vi "eval.vi"(8 "Environment in":T1, 9 "Expression in":T2) -> (2 "Environment out":T1, 3 "Expression out":T2)   [LabVIEW 2021]
uses:
  Expression.ctl
  ExpressionType.ctl
  Environment.ctl
  ClosureData.ctl
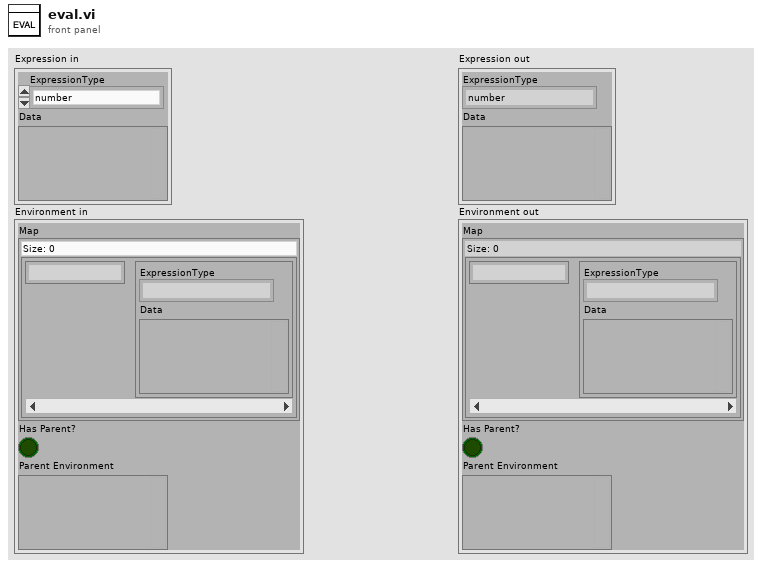
[diagram p1: front panel]
types:
  T1 = typedef "Environment.ctl" = cluster{"Map":map{string, T2}, "Has Parent?":bool, "Parent Environment":variant}
  T2 = typedef "Expression.ctl" = cluster{"ExpressionType":T3, "Data":variant}
  T3 = typedef "ExpressionType.ctl" = enum16{"number", "string", "symbol", "primitive", "list", "closure", "nil", "error"}
  T4 = typedef "ClosureData.ctl" = cluster{"arguments":string[], "code":T2}
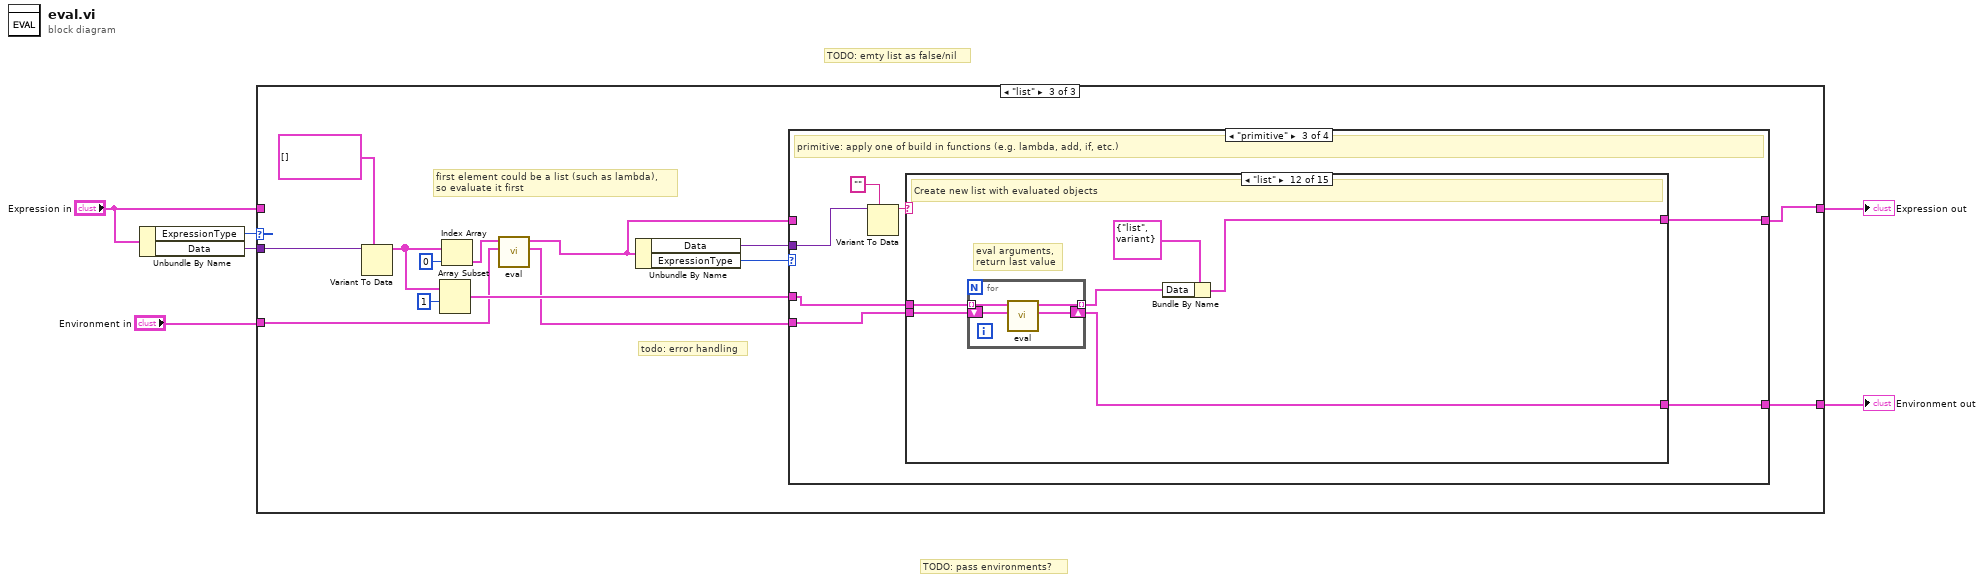
[diagram p0: block diagram]
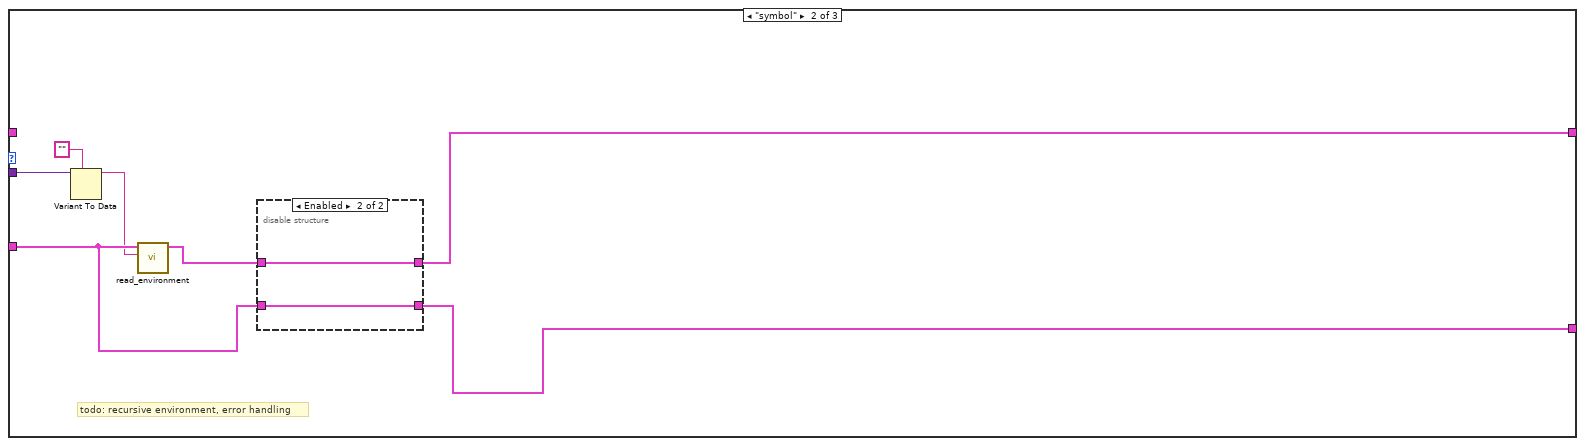
[diagram p3: hidden frame]
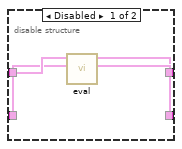
[diagram p4: hidden frame]
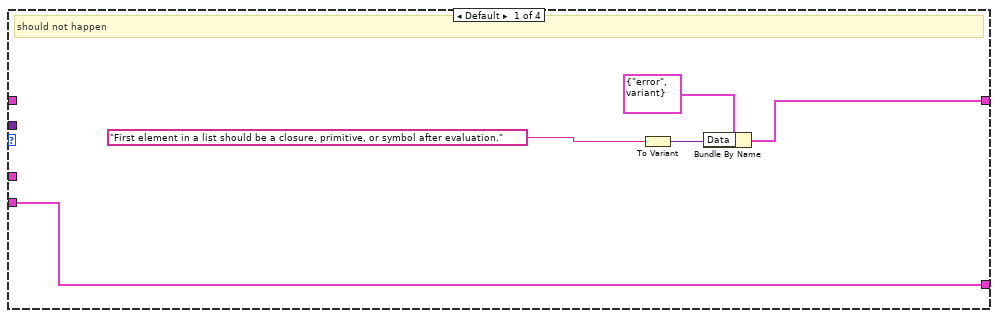
[diagram p5: hidden frame]
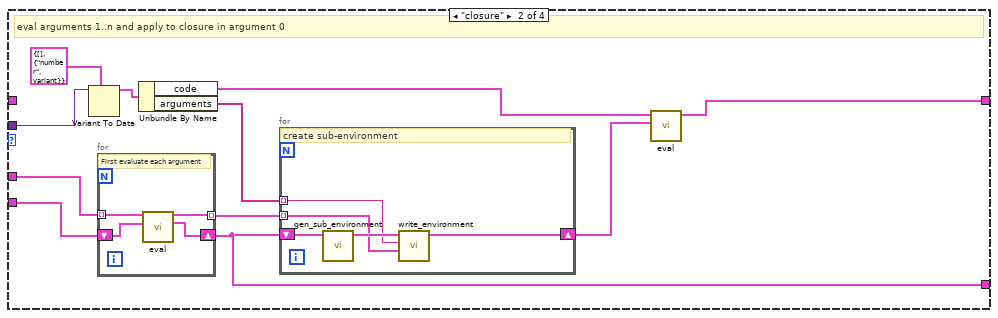
[diagram p6: hidden frame]
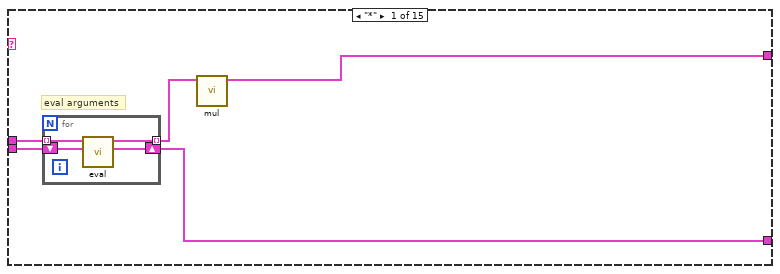
[diagram p7: hidden frame]
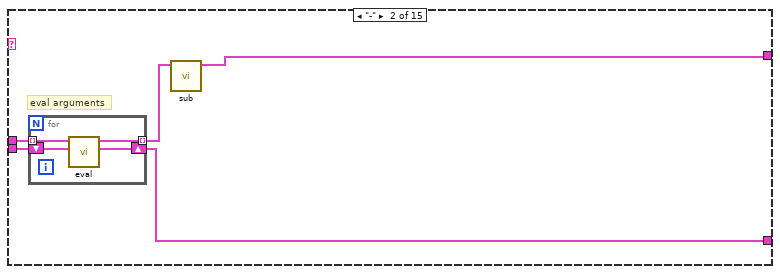
[diagram p8: hidden frame]
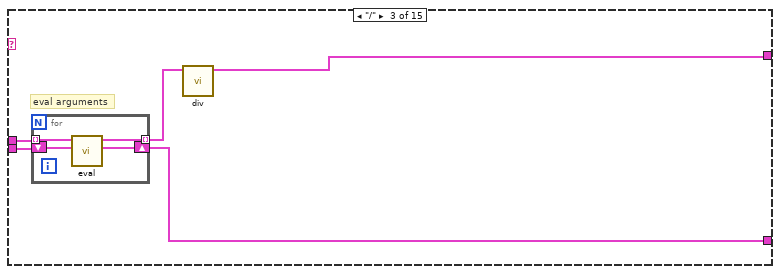
[diagram p9: hidden frame]
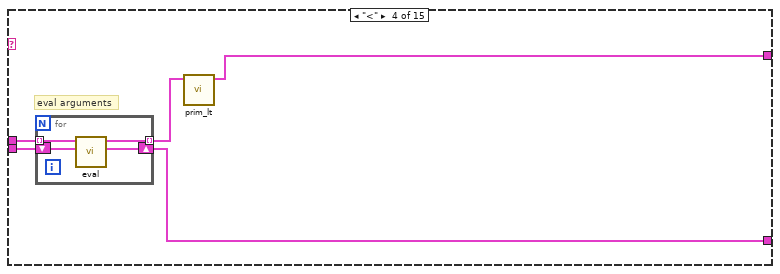
[diagram p10: hidden frame]
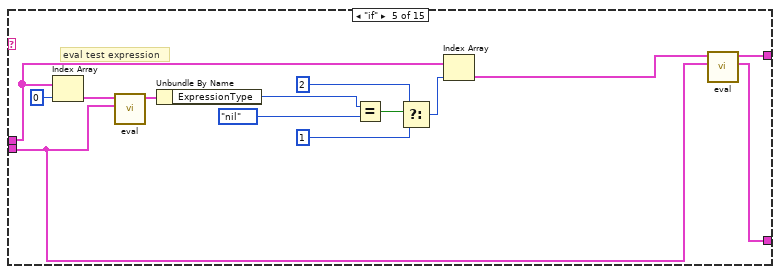
[diagram p11: hidden frame]
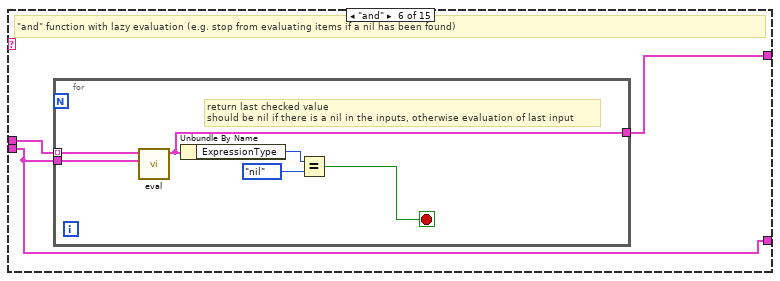
[diagram p12: hidden frame]
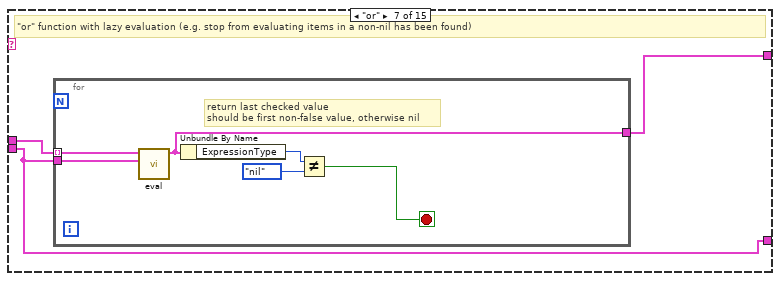
[diagram p13: hidden frame]
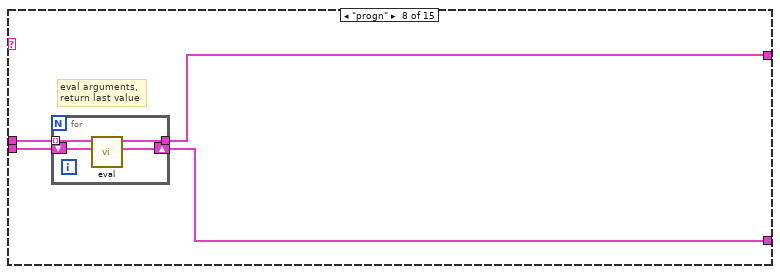
[diagram p14: hidden frame]
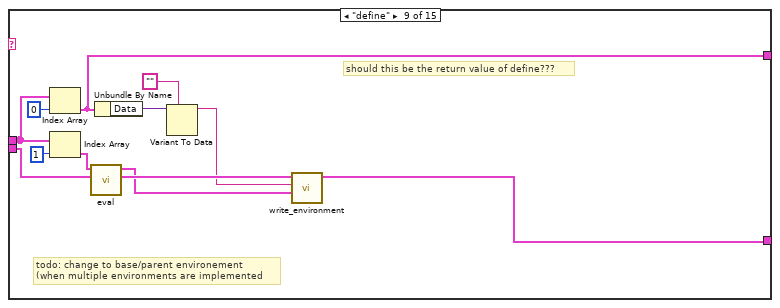
[diagram p15: hidden frame]
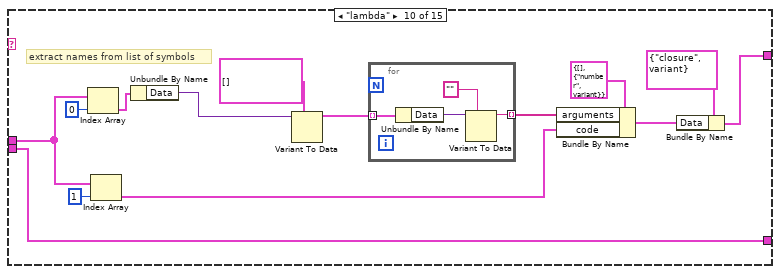
[diagram p16: hidden frame]
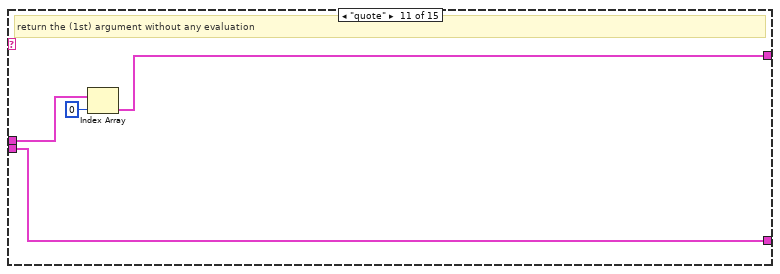
[diagram p17: hidden frame]
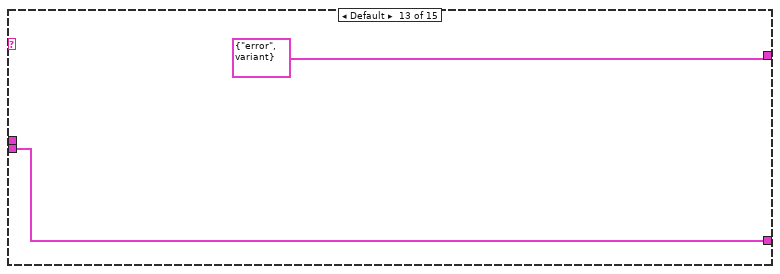
[diagram p18: hidden frame]
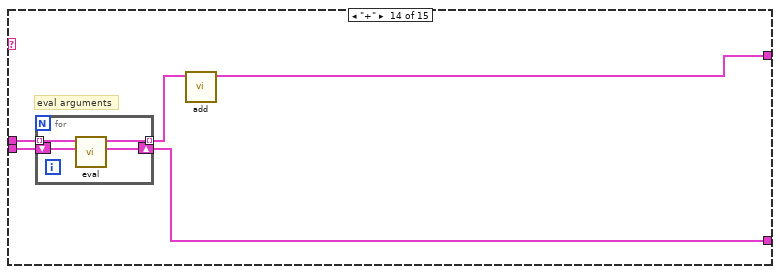
[diagram p19: hidden frame]
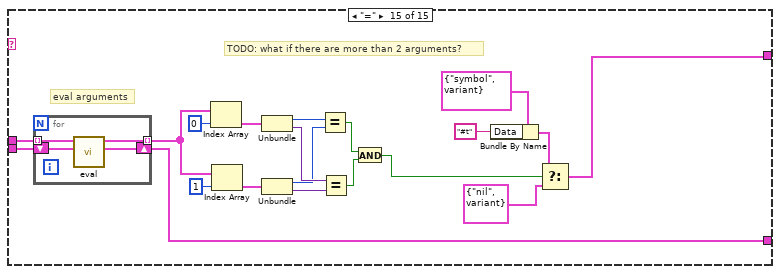
[diagram p20: hidden frame]
diagram:
  # "TODO: pass environments?"
  # "TODO: emty list as false/nil"
  n1 = Unbundle By Name("Expression in") -> ("ExpressionType"=w5:T3, "Data"=w3:variant)
  n2 = case shown="\"list\"" w5 {
    tunnel: "Expression in" -> [w8 _ _]
    tunnel: [w8 w12 w31] -> w4
    tunnel: "Environment in" -> [w7 w11 w23]
    tunnel: w3 -> [_ w15 w34]
    tunnel: [w7 w13 w22] -> w1
    frame "number", "string", "primitive", "closure".."error" {
    }
    frame "symbol" {
      # "todo: recursive environment, error handling"
      n3 = Variant To Data(type="", Variant=w15) -> (data=w9:string)  [unwired: 1 in, 1 out]
      n4 = call "read_environment.vi"("symbol"=w9, "Environment in"=w11) -> ("Expression"=w10:T2)  [unwired: 9 in]
      n5 = disable-structure shown="Enabled" {
        disable-tunnel: w10 -> [w19 w21]
        disable-tunnel: w11 -> [w18 w20]
        disable-tunnel: [w17 w20] -> w13
        disable-tunnel: [w16 w21] -> w12
        frame Disabled {
          n6 = call "eval.vi"("Environment in"=w18, "Expression in"=w19) -> ("Environment out"=w17:T1, "Expression out"=w16:T2)  [unwired: 6 in]
        }
        frame Enabled {
        }
      }
    }
    frame "list" {
      # "first element could be a list (such as lambda),\nso evaluate it first"
      # "todo: error handling"
      n7 = Variant To Data(type=T2[] [], Variant=w34) -> (data=w29:T2[])  [unwired: 1 in, 1 out]
      n8 = Array Subset(array=w29, index=1) -> (w28:T2[])  [unwired: 1 in]
      n9 = Index Array(array=w29, index=0) -> (element=w25:T2)
      n10 = call "eval.vi"("Environment in"=w23, "Expression in"=w25) -> ("Environment out"=w26:T1, "Expression out"=w24:T2)  [unwired: 6 in]
      n11 = Unbundle By Name(w24) -> ("Data"=w32:variant, "ExpressionType"=w27:T3)
      n12 = case shown="\"primitive\"" w27 {
        tunnel: w32 -> [_ w48 w66 w227]
        tunnel: w24 -> [_ _ _ _]
        tunnel: w26 -> [w40 w51 w62 w225]
        tunnel: [w36 w41 w64 w223] -> w31
        tunnel: w28 -> [_ w50 w63 _]
        tunnel: [w40 w44 w61 w225] -> w22
        frame Default {
          # "should not happen"
          n13 = To Variant(anything="First element in a list should be a closure, primitive, or symbol after evaluation.") -> (Variant=w38:variant)
          n14 = Bundle By Name(cluster=T2 {"ExpressionType"=enum."error", "Data"=variant} ("Expression out"), "Data"=w38) -> (w36:T2)
        }
        frame "closure" {
          # "eval arguments 1..n and apply to closure in argument 0"
          n15 = Variant To Data(type=T4 {"arguments"=[], "code"={"ExpressionType"=enum."number", "Data"=variant}} ("ClosureData"), Variant=w48) -> (data=w47:T4)  [unwired: 1 in, 1 out]
          n16 = for {
            shift-right: [w59] -> w44
            shift-left: w51 -> [w60]
            tunnel: w50 -> [w58] mode=indexing
            tunnel: [w57] -> w46 mode=indexing
            # "First evaluate each argument"
            n17 = call "eval.vi"("Environment in"=w60, "Expression in"=w58) -> ("Environment out"=w59:T1, "Expression out"=w57:T2)  [unwired: 6 in]
          }
          n18 = Unbundle By Name(w47) -> ("code"=w42:T2, "arguments"=w45:string[])
          n19 = for {
            tunnel: w46 -> [w52] mode=indexing
            tunnel: w45 -> [w53] mode=indexing
            shift-right: [w54] -> w43
            shift-left: w44 -> [w56]
            # "create sub-environment"
            n20 = call "gen_sub_environment.vi"("Environment in"=w56) -> ("Environment out"=w55:T1)  [unwired: 10 in]
            n21 = call "write_environment.vi"("Expression"=w52, "symbol"=w53, "Environment in"=w55) -> ("Environment out"=w54:T1)  [unwired: 8 in]
          }
          n22 = call "eval.vi"("Environment in"=w43, "Expression in"=w42) -> ("Expression out"=w41:T2)  [unwired: 6 in, 1 out]
        }
        frame "primitive" {
          # "primitive: apply one of build in functions (e.g. lambda, add, if, etc.)"
          n23 = Variant To Data(type="", Variant=w66) -> (data=w65:string)  [unwired: 1 in, 1 out]
          n24 = case shown="\"list\"" w65 {
            tunnel: [w72 w81 w90 w99 w109 w119 w128 w136 w148 w167 w174 w178 T2 {"ExpressionType"=enum."error", "Data"=variant} ("Expression 3") w194 w199] -> w64
            tunnel: w63 -> [w71 w80 w89 w98 w111 w120 w129 w139 w151 w160 w175 w183 _ w193 w218]
            tunnel: w62 -> [w70 w79 w88 w97 w110 w118 w127 w138 w155 w165 w177 w182 w188 w192 w217]
            tunnel: [w68 w77 w86 w95 w104 w118 w127 w137 w147 w165 w177 w179 w188 w190 w216] -> w61
            frame "*" {
              # "eval arguments"
              n25 = for {
                tunnel: w71 -> [w76] mode=indexing
                tunnel: [w74] -> w69 mode=indexing
                shift-right: [w73] -> w68
                shift-left: w70 -> [w75]
                n26 = call "eval.vi"("Environment in"=w75, "Expression in"=w76) -> ("Environment out"=w73:T1, "Expression out"=w74:T2)  [unwired: 6 in]
              }
              n27 = call "mul.vi"("arguments"=w69) -> ("Expression 3"=w72:T2)  [unwired: 10 in]
            }
            frame "-" {
              # "eval arguments"
              n28 = for {
                tunnel: w80 -> [w85] mode=indexing
                tunnel: [w83] -> w78 mode=indexing
                shift-right: [w82] -> w77
                shift-left: w79 -> [w84]
                n29 = call "eval.vi"("Environment in"=w84, "Expression in"=w85) -> ("Environment out"=w82:T1, "Expression out"=w83:T2)  [unwired: 6 in]
              }
              n30 = call "sub.vi"("arguments"=w78) -> ("Expression 3"=w81:T2)  [unwired: 10 in]
            }
            frame "/" {
              # "eval arguments"
              n31 = for {
                tunnel: w89 -> [w94] mode=indexing
                tunnel: [w92] -> w87 mode=indexing
                shift-right: [w91] -> w86
                shift-left: w88 -> [w93]
                n32 = call "eval.vi"("Environment in"=w93, "Expression in"=w94) -> ("Environment out"=w91:T1, "Expression out"=w92:T2)  [unwired: 6 in]
              }
              n33 = call "div.vi"("arguments"=w87) -> ("Expression 3"=w90:T2)  [unwired: 10 in]
            }
            frame "<" {
              # "eval arguments"
              n34 = for {
                tunnel: w98 -> [w103] mode=indexing
                tunnel: [w101] -> w96 mode=indexing
                shift-right: [w100] -> w95
                shift-left: w97 -> [w102]
                n35 = call "eval.vi"("Environment in"=w102, "Expression in"=w103) -> ("Environment out"=w100:T1, "Expression out"=w101:T2)  [unwired: 6 in]
              }
              n36 = call "prim_lt.vi"("arguments"=w96) -> ("Expression out"=w99:T2)  [unwired: 10 in]
            }
            frame "if" {
              # "eval test expression"
              n37 = Index Array(array=w111, index=0) -> (element=w116:T2)
              n38 = call "eval.vi"("Environment in"=w110, "Expression in"=w116) -> ("Expression out"=w108:T2)  [unwired: 6 in, 1 out]
              n39 = Unbundle By Name(w108) -> ("ExpressionType"=w107:T3)
              n40 = Equal?(x=w107, y=ExpressionType."nil") -> (x = y?=w105:bool)
              n41 = Select(t=2 ("index"), s=w105, f=1 ("index")) -> (s? t:f=w112:i32)
              n42 = Index Array(array=w111, index=w112) -> (element=w113:T2)
              n43 = call "eval.vi"("Environment in"=w110, "Expression in"=w113) -> ("Environment out"=w104:T1, "Expression out"=w109:T2)  [unwired: 6 in]
            }
            frame "and" {
              # "\"and\" function with lazy evaluation (e.g. stop from evaluating items if a nil has been found)"
              n44 = for {
                tunnel: w118 -> [w124]
                tunnel: w120 -> [w123] mode=indexing
                tunnel: [w121] -> w119
                stop <- w122 stop-if-true
                # "return last checked value\nshould be nil if there is a nil in the inputs, otherwise evaluation of last input"
                n45 = call "eval.vi"("Environment in"=w124, "Expression in"=w123) -> ("Expression out"=w121:T2)  [unwired: 6 in, 1 out]
                n46 = Unbundle By Name(w121) -> ("ExpressionType"=w126:T3)
                n47 = Equal?(x=w126, y=ExpressionType."nil") -> (x = y?=w122:bool)
              }
            }
            frame "or" {
              # "\"or\" function with lazy evaluation (e.g. stop from evaluating items in a non-nil has been found)"
              n48 = for {
                tunnel: w127 -> [w133]
                tunnel: w129 -> [w132] mode=indexing
                tunnel: [w130] -> w128
                stop <- w131 stop-if-true
                # "return last checked value\nshould be first non-false value, otherwise nil"
                n49 = call "eval.vi"("Environment in"=w133, "Expression in"=w132) -> ("Expression out"=w130:T2)  [unwired: 6 in, 1 out]
                n50 = Unbundle By Name(w130) -> ("ExpressionType"=w135:T3)
                n51 = Not Equal?(x=w135, y=ExpressionType."nil") -> (x != y?=w131:bool)
              }
            }
            frame "progn" {
              # "eval arguments,\nreturn last value"
              n52 = for {
                tunnel: w139 -> [w143] mode=indexing
                tunnel: [w141] -> w136
                shift-right: [w140] -> w137
                shift-left: w138 -> [w142]
                n53 = call "eval.vi"("Environment in"=w142, "Expression in"=w143) -> ("Environment out"=w140:T1, "Expression out"=w141:T2)  [unwired: 6 in]
              }
            }
            frame "define" {
              # "todo: change to base/parent environement\n(when multiple environments are implemented"
              # "should this be the return value of define???"
              n54 = Index Array(array=w151, index=0) -> (element=w148:T2)
              n55 = Index Array(array=w151, index=1) -> (element=w153:T2)
              n56 = call "eval.vi"("Environment in"=w155, "Expression in"=w153) -> ("Environment out"=w146:T1, "Expression out"=w145:T2)  [unwired: 6 in]
              n57 = Unbundle By Name(w148) -> ("Data"=w150:variant)
              n58 = Variant To Data(type="", Variant=w150) -> (data=w144:string)  [unwired: 1 in, 1 out]
              n59 = call "write_environment.vi"("Expression"=w145, "symbol"=w144, "Environment in"=w146) -> ("Environment out"=w147:T1)  [unwired: 8 in]
            }
            frame "lambda" {
              # "extract names from list of symbols"
              n60 = Index Array(array=w160, index=0) -> (element=w159:T2)
              n61 = Index Array(array=w160, index=1) -> (element=w162:T2)
              n62 = Unbundle By Name(w159) -> ("Data"=w157:variant)
              n63 = Variant To Data(type=T2[] [], Variant=w157) -> (data=w156:T2[])  [unwired: 1 in, 1 out]
              n64 = for {
                tunnel: w156 -> [w173] mode=indexing
                tunnel: [w170] -> w164 mode=indexing
                n65 = Unbundle By Name(w173) -> ("Data"=w172:variant)
                n66 = Variant To Data(type="", Variant=w172) -> (data=w170:string)  [unwired: 1 in, 1 out]
              }
              n67 = Bundle By Name(cluster=T4 {"arguments"=[], "code"={"ExpressionType"=enum."number", "Data"=variant}} ("ClosureData"), "arguments"=w164, "code"=w162) -> (w166:T4)
              n68 = Bundle By Name(cluster=T2 {"ExpressionType"=enum."closure", "Data"=variant} ("Expression 3"), "Data"=w166) -> (w167:T2)
            }
            frame "quote" {
              # "return the (1st) argument without any evaluation"
              n69 = Index Array(array=w175, index=0) -> (element=w174:T2)
            }
            frame "list" {
              # "eval arguments,\nreturn last value"
              # "Create new list with evaluated objects"
              n70 = for {
                tunnel: w183 -> [w187] mode=indexing
                tunnel: [w185] -> w180 mode=indexing
                shift-right: [w184] -> w179
                shift-left: w182 -> [w186]
                n71 = call "eval.vi"("Environment in"=w186, "Expression in"=w187) -> ("Environment out"=w184:T1, "Expression out"=w185:T2)  [unwired: 6 in]
              }
              n72 = Bundle By Name(cluster=T2 {"ExpressionType"=enum."list", "Data"=variant} ("Expression out"), "Data"=w180) -> (w178:T2)
            }
            frame Default {
            }
            frame "+" {
              # "eval arguments"
              n73 = for {
                tunnel: w193 -> [w198] mode=indexing
                tunnel: [w196] -> w191 mode=indexing
                shift-right: [w195] -> w190
                shift-left: w192 -> [w197]
                n74 = call "eval.vi"("Environment in"=w197, "Expression in"=w198) -> ("Environment out"=w195:T1, "Expression out"=w196:T2)  [unwired: 6 in]
              }
              n75 = call "add.vi"("arguments"=w191) -> ("Expression 3"=w194:T2)  [unwired: 10 in]
            }
            frame "=" {
              # "TODO: what if there are more than 2 arguments?"
              # "eval arguments"
              n76 = for {
                tunnel: w218 -> [w222] mode=indexing
                tunnel: [w220] -> w211 mode=indexing
                shift-right: [w219] -> w216
                shift-left: w217 -> [w221]
                n77 = call "eval.vi"("Environment in"=w221, "Expression in"=w222) -> ("Environment out"=w219:T1, "Expression out"=w220:T2)  [unwired: 6 in]
              }
              n78 = Index Array(array=w211, index=0) -> (element=w208:T2)
              n79 = Index Array(array=w211, index=1) -> (element=w207:T2)
              n80 = Unbundle(w208) -> ("ExpressionType"=w206:T3, "Data"=w204:variant)
              n81 = Unbundle(w207) -> ("ExpressionType"=w203:T3, "Data"=w205:variant)
              n82 = Equal?(x=w206, y=w203) -> (x = y?=w202:bool)
              n83 = Equal?(x=w204, y=w205) -> (x = y?=w201:bool)
              n84 = And(x=w202, y=w201) -> (x .and. y?=w200:bool)
              n85 = Bundle By Name(cluster=T2 {"ExpressionType"=enum."symbol", "Data"=variant} ("Expression 3"), "Data"="#t") -> (w215:T2)
              n86 = Select(t=w215, s=w200, f=T2 {"ExpressionType"=enum."nil", "Data"=variant} ("Expression 3")) -> (s? t:f=w199:T2)
            }
          }
        }
        frame "symbol" {
          n87 = Variant To Data(type="", Variant=w227) -> (data=w224:string)  [unwired: 1 in, 1 out]
          n88 = call "read_environment.vi"("symbol"=w224, "Environment in"=w225) -> ("Expression"=w223:T2)  [unwired: 9 in]
        }
      }
    }
  }
  "Expression out" <- w4
  "Environment out" <- w1
